vi "test objects.vi"() -> ()   [LabVIEW 2025]
uses:
  Classes/Processor/Processor.lvclass
panel:
  out "error out":errorcluster
  out "data":dbl
  out "Processor out":refnum<class "Processor.lvclass">
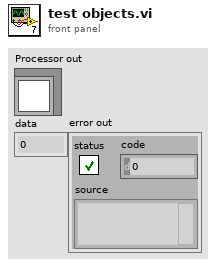
[diagram p1: front panel]
types:
  T1 = cluster{"Thermal Tape":refnum<class "Processor.lvclass">, "Thermocouples":refnum<class "Processor.lvclass">}
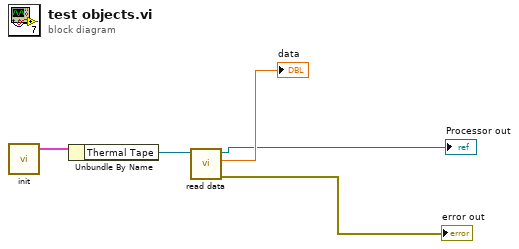
[diagram p0: block diagram]
diagram:
  n1 = call "init.vi"() -> ("objects"=w5:T1)  [unwired: 10 in, 1 out]
  n2 = Unbundle By Name(w5) -> ("Thermal Tape"=w4:refnum<class "Processor.lvclass">)
  n3 = call-dynamic "read data.vi"("Processor in"=w4) -> ("error out"=→"error out":errorcluster, "data"=→"data":dbl, "Processor out"=→"Processor out":refnum<class "Processor.lvclass">)  [unwired: 8 in]
